vi "Add Space to Prefix.vi"(11 "Target File Prefix in":string) -> (3 "Target File Prefix out":string)   [LabVIEW 2016, in "NI_NPW_Project Copying.lvlib"]
uses:
  <resource>/dialog/NewProjectWizard/Project Copying/NI_NPW_Project Copying.lvlib
  <resource>/dialog/lvconfig.llb/LV Config Read Boolean.vi
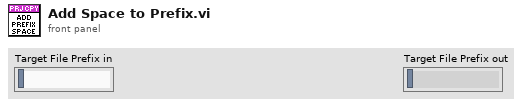
[diagram p1: front panel]
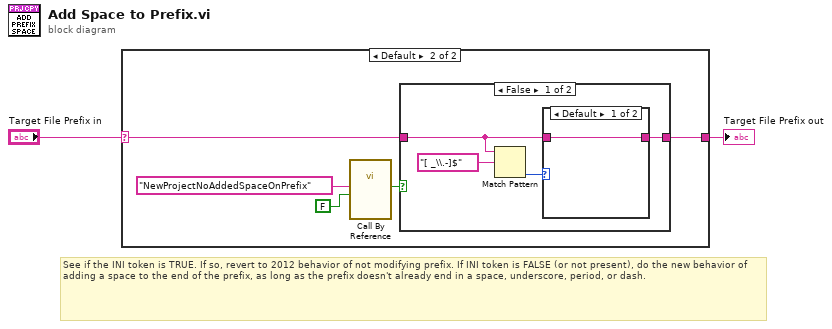
[diagram p0: block diagram]
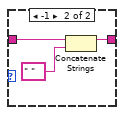
[diagram p3: hidden frame]
diagram:
  # "See if the INI token is TRUE. If so, revert to 2012 behavior of not modifying prefix. If INI token is FALSE (or not present), do the new behavior of adding a space to the end of the prefix, as long as the prefix doesn't already end in a space, underscore, period, or dash."
  n1 = case shown="Default" "Target File Prefix in" {
    selector: "Target File Prefix in" -> [w3 w4]
    tunnel: [w3 w8] -> w2
    frame "" {
      # "Don't edit the prefix if it is blank"
    }
    frame Default {
      n2 = call-by-ref "?"("default value"=FALSE, "key"="NewProjectNoAddedSpaceOnPrefix") -> ("value"=w5:bool)  [unwired: 5 in, 4 out]
      n3 = case shown="False" w5 {
        tunnel: w4 -> [w10 w17]
        tunnel: [w9 w17] -> w8
        frame False {
          n4 = Match Pattern(string=w10, regular expression="[ _\\.-]$") -> (offset past match=w11:i32)  [unwired: 1 in, 3 out]
          n5 = case shown="Default" w11 {
            tunnel: w10 -> [w13 w16]
            tunnel: [w13 w15] -> w9
            frame Default {
            }
            frame -1 {
              n6 = Concatenate Strings(w16, " ") -> (w15:string)
            }
          }
        }
        frame True {
        }
      }
    }
  }
  "Target File Prefix out" <- w2
